vi "Configure Monitor Scan.vi"(0 "VISA resource name":refnum<visa-resource-name>, 1 "Monitor Channel (Empty)":string, 5 "Enable Monitor Scan (False)":bool, 9 "Number of Channels (2)":i32=2, 11 "error in (no error)":errorcluster) -> (4 "VISA resource name out":refnum<visa-resource-name>, 15 "error out":errorcluster={"status"=FALSE, "code"=1, "source"=""})   [LabVIEW 2020, in "Keithley 27XX.lvlib"]
doc: "This VI enables or disables a monitor scan, sets the number of channels to scan, and sets the channel to use as the monitor channel."
uses:
  <instrlib>/Keithley 27XX/Keithley 27XX.lvlib
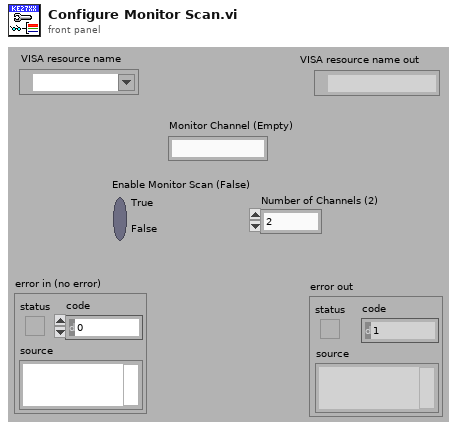
[diagram p1: front panel]
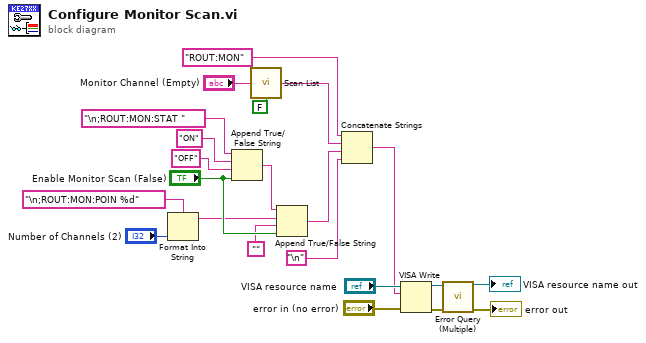
[diagram p0: block diagram]
diagram:
  n1 = Format Into String(format string="\n;ROUT:MON:POIN %d", "Number of Channels (2)") -> (resulting string=w7:string)  [unwired: 2 in, 1 out]
  n2 = Append True/False String(1:"Enable Monitor Scan (False)", 2:"OFF" ("false string"), 3:"ON" ("true string"), 4:"\n;ROUT:MON:STAT ") -> (0:w14:string)
  n3 = call <instrlib>:"Scan List.vi"("Add Comma (True)"=FALSE ("Comma? (True)"), "Scan List (Empty)"="Monitor Channel (Empty)") -> ("Scan List Out"=w17:string)  [unwired: 13 in]
  n4 = Append True/False String(1:"Enable Monitor Scan (False)", 2:"", 3:w7, 4:w14) -> (0:w13:string)
  n5 = Concatenate Strings("ROUT:MON", w17, w13, "\n") -> (w10:string)
  n6 = VISA Write(VISA resource name="VISA resource name", write buffer=w10, error in (no error)="error in (no error)") -> (VISA resource name out=w5:refnum<visa-resource-name>, error out=w4:errorcluster)  [unwired: 1 out]
  n7 = call <instrlib>:"Error Query (Multiple).vi"("VISA resource name"=w5, "error in (no error)"=w4) -> ("VISA resource name out"=→"VISA resource name out":refnum<visa-resource-name>, "error out"=→"error out":errorcluster)  [unwired: 10 in, 2 out]
